vi "PicoScope3000aExampleRapidBlockBulkMSO.vi"() -> ()   [LabVIEW 2009]
uses:
  <vilib>/Waveform/DWDTOps.llb/DWDT Analog to Digital.vi
panel:
  in  "Channel A Trigger Properties":T1 {"Direction" items=["Above / Inside", "Below / Outside", "Rising / Enter", "Falling / Exit", "Rising or Falling / Enter or Exit", "Above Lower", "Below Lower", "Rising Lower", "Falling Lower", "Positive Runt", "Negative Runt"]; "Threshold Mode" items=["Level", "Window"]}
  in  "Number of Segments":u32
  out "USB Powered":bool
  out "USB 3.0 device on non-USB 3.0 Port":bool
  in  "Rapid Block Bulk\nAcquisition Settings":T2 {"Down Sample Ratio" min=1 step=1; "Down-Sample Mode" items=["None", "Aggregate", "Decimate", "Average"]}
  in  "Channel A Settings":T3 {"Range" items=["10 mV", "20 mV", "50 mV", "100 mV", "200 mV", "500 mV", "1 V", "2 V", "5 V", "10 V", "20 V", "50 V ", "100 V"]; "Coupling" items=["AC", "DC"]}
  in  "Trigger Conditions":T4 {"Condition Logic" items=["AND", "OR", "XOR"]}
  in  "Digital Port  0":T5 {"Direction Channel 7" items=["Don't Care", "Low", "High", "Rising", "Falling"]; "Direction Channel 6" items=["Don't Care", "Low", "High", "Rising", "Falling"]; "Direction Channel 5" items=["Don't Care", "Low", "High", "Rising", "Falling"]; "Direction Channel 4" items=["Don't Care", "Low", "High", "Rising", "Falling"]; "Direction Channel 3" items=["Don't Care", "Low", "High", "Rising", "Falling"]; "Direction Channel 2" items=["Don't Care", "Low", "High", "Rising", "Falling"]; "Direction Channel 1" items=["Don't Care", "Low", "High", "Rising", "Falling"]; "Direction Channel 0" items=["Don't Care", "Low", "High", "Rising", "Falling"]}
  out "Port 0 Digital Waveform Graph":digitalwaveform(graph)
  in  "Port 0 Settings":cluster{"Enabled":bool, "Logic Level":u16} {"Logic Level" items=["1.5V TTL", "2.5V CMOS"]}
  out "Capture Complete":bool
  in  "Run":bool
  out "Channel A":i16[](graph)
  in  "Capture Index":i16 min=0
  in  "stop":bool
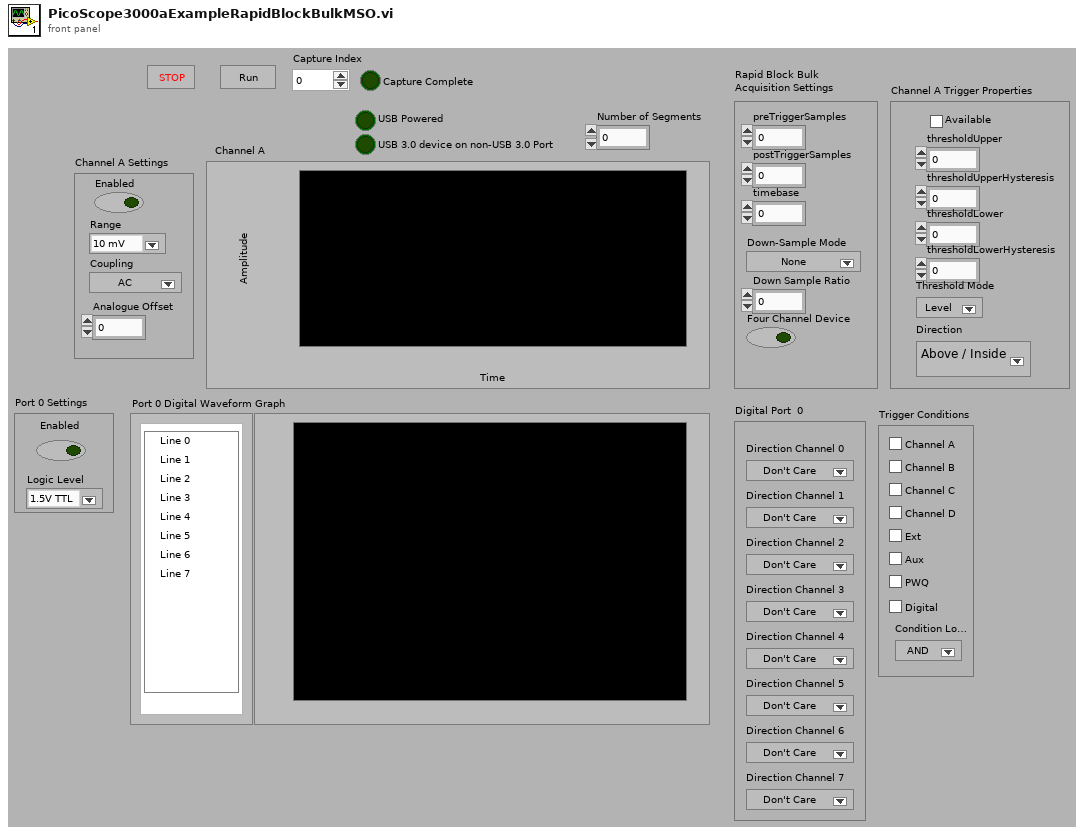
[diagram p1: front panel]
types:
  T1 = cluster{"thresholdUpper":i16, "thresholdUpperHysteresis":u16, "thresholdLower":i16, "thresholdLowerHysteresis":u16, "Threshold Mode":i32, "Direction":i32, "Available":bool}
  T2 = cluster{"preTriggerSamples":u32, "postTriggerSamples":u32, "timebase":u32, "Down-Sample Mode":i32, "Down Sample Ratio":u32, "Four Channel Device":bool}
  T3 = cluster{"Enabled":bool, "Coupling":u32, "Range":u32, "Analogue Offset":sgl}
  T4 = cluster{"Channel A":bool, "Channel B":bool, "Channel C":bool, "Channel D":bool, "Aux":bool, "PWQ":bool, "Condition Logic":u16, "Ext":bool, "Digital":bool}
  T5 = cluster{"Direction Channel 0":u16, "Direction Channel 1":u16, "Direction Channel 2":u16, "Direction Channel 3":u16, "Direction Channel 4":u16, "Direction Channel 5":u16, "Direction Channel 6":u16, "Direction Channel 7":u16}
  T6 = cluster{"Driver Version":string, "USB Version":string, "Hardware":string, "Variant":string, "Batch and Serial":string, "Cal Date":string, "Kernel Version":string, "Digital HW Version":string, "Analogue HW Version":string, "MSO":bool, "Number of channels":i16}
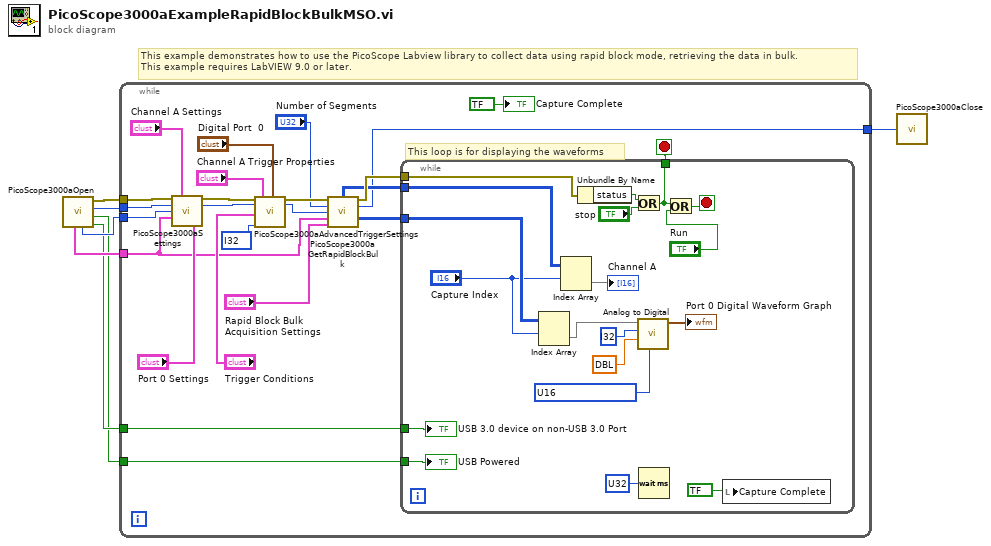
[diagram p0: block diagram]
diagram:
  # "This example demonstrates how to use the PicoScope Labview library to collect data using rapid block mode, retrieving the data in bulk.\nThis example requires LabVIEW 9.0 or later."
  n1 = call "PicoScope3000aOpen.vi"() -> ("USB 3.0 device on non-USB 3.0 Port"=w2:bool, "USB Powered"=w1:bool, "handle"=w5:i16, "error out"=w6:errorcluster, "Max ADC value"=w3:i16, "Device Info"=w4:T6)  [unwired: 6 in]
  n2 = while {
    tunnel: [w27] -> w7
    tunnel: w6 -> [w26]
    tunnel: w5 -> [w25]
    tunnel: w4 -> [w9]
    tunnel: w3 -> [w13]
    tunnel: w2 -> [w12]
    tunnel: w1 -> [w11]
    stop <- w31 stop-if-true
    # "This loop is for displaying the waveforms"
    n3 = call "PicoScope3000aSettings.vi"("error in"=w26, "Channel A Settings"="Channel A Settings", "Port 0 Settings"="Port 0 Settings", "handle in"=w25, "Max_adc"=w13, "Device Info"=w9) -> ("error out"=w20:errorcluster, "handle out"=w19:i16)  [unwired: 7 in, 1 out]
    n4 = call "PicoScope3000aAdvancedTriggerSettings.vi"("error in"=w20, "handle in"=w19, "Trigger Conditions"="Trigger Conditions", "Auto Trigger (ms)"=i32 ?, "Channel A Trigger Properties"="Channel A Trigger Properties", "Digital Port  0"="Digital Port  0") -> ("error out"=w22:errorcluster, "handle out"=w21:i16)  [unwired: 12 in]
    n5 = call "PicoScope3000aGetRapidBlockBulk.vi"("error in"=w22, "Number of Segments"="Number of Segments", "handle in"=w21, "Device Info"=w9, "Rapid Block Bulk Acquisition Settings"="Rapid Block Bulk\nAcquisition Settings") -> ("Channel A Buffer"=w28:i16[][], "error out"=w29:errorcluster, "handle out"=w27:i16, "Port 0 Buffer"=w23:i16[][])  [unwired: 2 in, 5 out]
    n6 = while {
      tunnel: [w49] -> w31
      tunnel: w28 -> [w35]
      tunnel: w29 -> [w44]
      tunnel: w23 -> [w38]
      tunnel: w12 -> [w33]
      tunnel: w11 -> [w32]
      stop <- w48 stop-if-true
      w39 = u16 ? items=["unsigned binary", "offset binary", "2's complement"] ("data format (offset binary)")
      n7 = Index Array(array=w38, index (row)="Capture Index") -> (element=w37:i16[])  [unwired: 1 in]
      n8 = Index Array(array=w35, index (row)="Capture Index") -> (element=→"Channel A":i16[])  [unwired: 1 in]
      n9 = Unbundle By Name(w44) -> ("status"=w43:bool)
      n10 = Or(x=w43, y="stop") -> (x .or. y?=w49:bool)
      n11 = call-poly <vilib>:"Analog to Digital.vi"("data format (offset binary)"=w39, "full-scale range (pk-pk)"=dbl ?, "resolution (16 bit)"=i32 ?, "analog waveform"=w37) -> ("digital waveform"=→"Port 0 Digital Waveform Graph":digitalwaveform)  [unwired: 4 in, 3 out]
      n12 = Wait (ms)(milliseconds to wait=u32 ?) -> ()  [unwired: 1 out]
      n13 = Or(x=w49, y="Run") -> (x .or. y?=w48:bool)
      n14 = local write "Capture Complete"(bool ? ("Capture Complete")) -> ()
      "USB 3.0 device on non-USB 3.0 Port" <- w33
      "USB Powered" <- w32
    }
    "Capture Complete" <- bool ? ("Capture Complete")
  }
  n15 = call "PicoScope3000aClose.vi"("handle"=w7) -> ()
